vi "Execute.vi"(8 "error in (no error)":errorcluster, 11 "Test Step in":refnum<class "Test Step.lvclass">) -> (0 "error out":errorcluster, 2 "Test Result":refnum<class "Test Result.lvclass">, 3 "Test Step out":refnum<class "Test Step.lvclass">)   [LabVIEW 2021, in "Sequence Engine.lvlib" / "Test Step.lvclass"]
uses:
  Test Step.lvclass
  Test Step.lvclass/Test Step.ctl
  Test Result/Test Result.lvclass
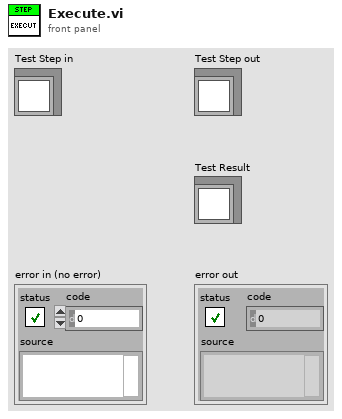
[diagram p1: front panel]
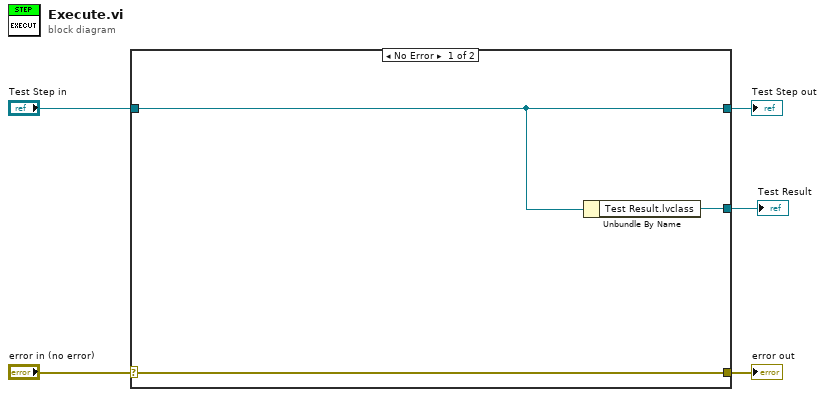
[diagram p0: block diagram]
diagram:
  n1 = case shown="No Error" "error in (no error)" {
    selector: "error in (no error)" -> [w8 w10]
    tunnel: [w8 w10] -> w4
    tunnel: [w7 w9] -> w2
    tunnel: "Test Step in" -> [w7 w9]
    tunnel: [w6 _] -> w1
    frame No Error {
      n2 = Unbundle By Name(w7) -> ("Test Result.lvclass"=w6:refnum<class "Test Result.lvclass">)
    }
    frame Error {
    }
  }
  "error out" <- w4
  "Test Step out" <- w2
  "Test Result" <- w1
